vi "McP789A-INIT-v0.49.vi"(5 "error in (no error)":errorcluster) -> (0 "error out":errorcluster={"status"=TRUE, "code"=65, "source"="McP Timeout"}, 1 "Current Stepper Position":i32, 2 "Scan Velocity (steps/sec)":i32=42372, 3 "MCP CounterReading":dbl=666.0 format="%.2f")   [LabVIEW 2020]
doc: "Open the serial port, initialize the McP 789A-3 controller. Also load the counter position through file. Output scan velocity and counter position.\n\nThe serial port is a global variable. The scan velocity is also a global variable, and is assaigned by McP Status VI called by this VI."
uses:
  Globals and TypeDefs/Global Varibal Control.vi
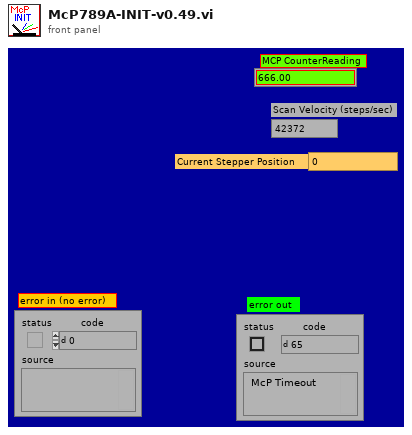
[diagram p1: front panel]
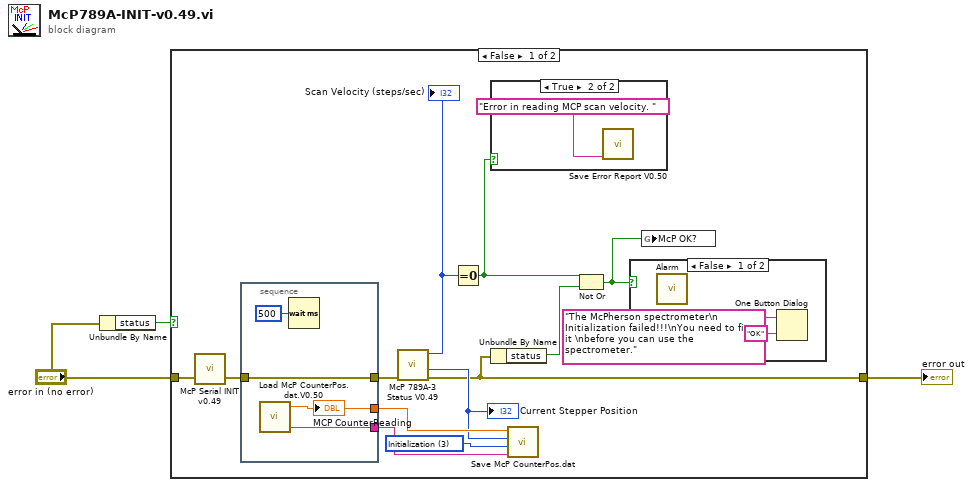
[diagram p0: block diagram]
diagram:
  n1 = Unbundle By Name("error in (no error)") -> ("status"=w1:bool)
  n2 = case shown="False" w1 {
    tunnel: "error in (no error)" -> [w15 w23]
    tunnel: [w7 w23] -> w2
    frame False {
      w10 = u16 3 items=["Moving", "Calibration", "Key in", "Initialization"] ("Set Method")
      n3 = call "McP Serial INIT v0.49.vi"("error in (no error)"=w15) -> ("Error out"=w14:errorcluster)  [unwired: 1 in, 1 out]
      n4 = stacked-sequence {
        tunnel: [w20] -> w13
        tunnel: w14 -> [w20]
        tunnel: [w19] -> w12
        tunnel: [w18] -> w9
        frame #0 {
          n5 = call "Load McP CounterPos.dat.V0.50.vi"() -> ("Counter Position"=w19:dbl, "Last Calibration Date"=w18:string)  [unwired: 1 in, 1 out]
          "MCP CounterReading" <- w19
          n6 = Wait (ms)(milliseconds to wait=u32 500) -> ()  [unwired: 1 out]
        }
      }
      n7 = call "McP 789A-3 Status V0.49.vi"("error in (no error)"=w13) -> ("error out"=w7:errorcluster, "CurrentPosition"=w11:i32, "Velocity (Steps/s)"=w8:i32)  [unwired: 7 in, 1 out]
      "Scan Velocity (steps/sec)" <- w8
      "Current Stepper Position" <- w11
      n8 = Equal To 0?(x=w8) -> (x = 0?=w5:bool)
      n9 = case shown="True" w5 {
        frame False {
        }
        frame True {
          n10 = call "Save Error Report V0.50.vi"("Error Message"="Error in reading MCP scan velocity. " ("message")) -> ()  [unwired: 5 in, 1 out]
        }
      }
      n11 = Unbundle By Name(w7) -> ("status"=w4:bool)
      n12 = call "Save McP CounterPos.dat.vi"("Last Calibration Date"=w9, "Set Method"=w10, "McP Stepper Position"=w11, "McP Counter Position"=w12) -> ()  [unwired: 2 in, 1 out]
      n13 = Not Or(1:w4, 2:w5) -> (0:w6:bool)
      n14 = case shown="False" w6 {
        frame False {
          n15 = call "Alarm.vi"() -> ()  [unwired: 4 in]
          n16 = One Button Dialog(message="The McPherson spectrometer\n Initialization failed!!!\nYou need to fix it \nbefore you can use the spectrometer.", button name ("OK")="OK") -> ()  [unwired: 1 out]
        }
        frame True {
        }
      }
      n17 = global write "Global Varibal Control.vi" "McP OK?"(w6) -> ()
    }
    frame True {
    }
  }
  "error out" <- w2
